vi "Is_Remote_loaded.vi"(0 "Sub VI to call":string) -> ()   [LabVIEW 2010]
uses:
  Globals/Dynamic_call_global.ph.vi
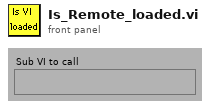
[diagram p1: front panel]
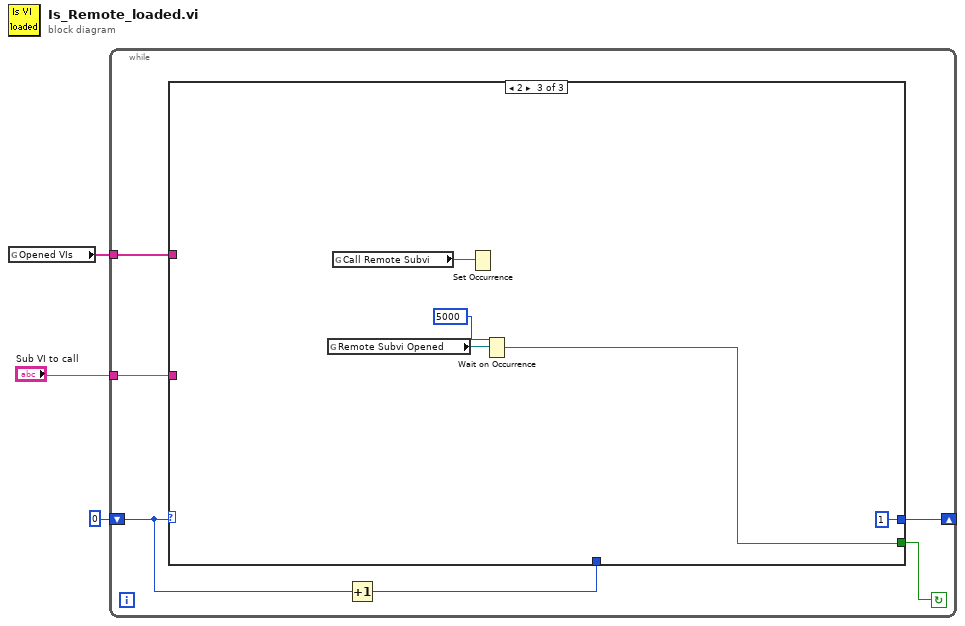
[diagram p0: block diagram]
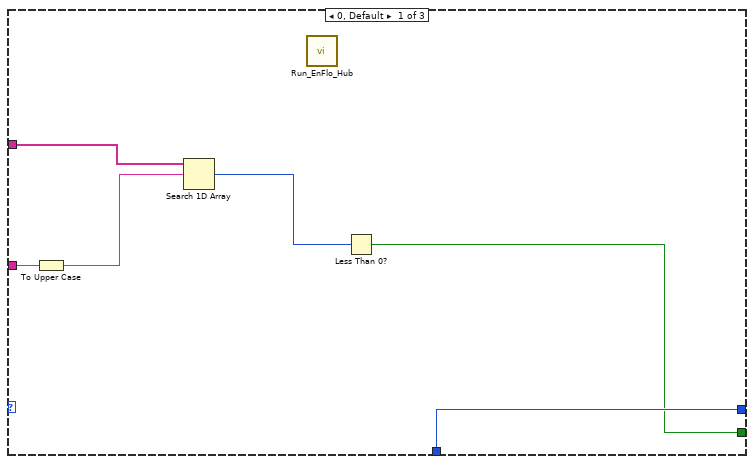
[diagram p2: hidden frame]
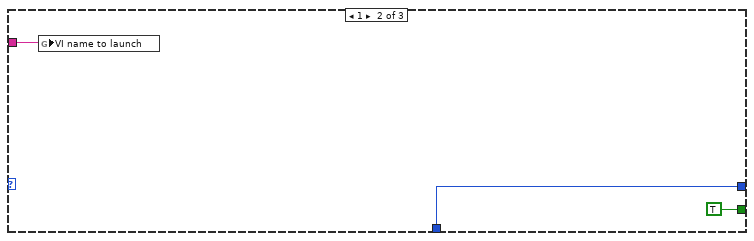
[diagram p3: hidden frame]
diagram:
  n1 = global read "Dynamic_call_global.ph.vi" "Opened VIs"() -> (w2:string[])
  n2 = while {
    tunnel: w2 -> [w5]
    tunnel: "Sub VI to call" -> [w6]
    shift-left: 0 -> [w9]
    shift-right: [w8] -> _
    stop <- w4 continue-if-true
    n3 = Increment(x=w9) -> (x+1=w7:i32)
    n4 = case shown="2" w9 {
      tunnel: [w13 w16 1] -> w8
      tunnel: w7 -> [w13 w16 _]
      tunnel: w6 -> [w11 w17 _]
      tunnel: w5 -> [w15 _ _]
      tunnel: [w12 TRUE w20] -> w4
      frame 0, Default {
        n5 = To Upper Case(1:w11) -> (0:w10:string)
        n6 = Search 1D Array(1D array=w15, element=w10) -> (index of element=w14:i32)  [unwired: 1 out]
        n7 = call "Run_EnFlo_Hub.vi"() -> ()  [unwired: 8 out]
        n8 = Less Than 0?(x=w14) -> (x < 0?=w12:bool)
      }
      frame 1 {
        n9 = global write "Dynamic_call_global.ph.vi" "VI name to launch"(w17) -> ()
      }
      frame 2 {
        n10 = global read "Dynamic_call_global.ph.vi" "Remote Subvi Opened"() -> (w23:refnum<k4>)
        n11 = global read "Dynamic_call_global.ph.vi" "Call Remote Subvi"() -> (w22:refnum<k4>)
        n12 = Set Occurrence(w22) -> ()
        n13 = Wait on Occurrence(2:w23, 3:5000 ("ms timeout (-1)")) -> (0:w20:bool)  [unwired: 1 out]
      }
    }
  }
